vi "Agilent 34401 Read Single Measurement.vi"() -> ()   [LabVIEW 2013]
doc: "This example shows how to configure a measurement and take a single reading."
uses:
  <vilib>/Utility/error.llb/DialogType.ctl
  <instrlib>/Agilent 34401/Public/Data/Read (Single Point).vi
  <instrlib>/Agilent 34401/Agilent 34401.lvlib
panel:
  in  "Function (0: DC Voltage)":u16(ring) items=["DC Voltage", "AC Voltage", "2 - Wire Resistance", "4 - Wire Resistance", "DC Current", "AC Current", "Frequency", "Period", "Continuity", "Diode Checking", "VDC:VDC Ratio", "Temperature", "Capacitance"]
  in  "Enable Auto Range (T: Enable)":bool=TRUE
  in  "Manual Resolution (5.5 Digits)":dbl(ring)=5.5 items=["4.5"=4.5, "5.5"=5.5, "6.5"=6.5]
  in  "Manual Range (1.00)":dbl=1.0 format="%_3f"
  in  "Serial Configuration":T1={"Baud Rate"=9600, "Parity"=2, "Data Bits"=7} {"Data Bits" items=["7"=7, "8"=8]; "Parity" items=["None", "Odd", "Even"]; "Baud Rate" items=["300"=300, "600"=600, "1200"=1200, "2400"=2400, "4800"=4800, "9600"=9600, "19200"=19200]}
  out "Measurement":dbl
  in  "VISA resource name":refnum<visa-resource-name>
  # "(c) 2005-2008 National Instruments.  ALL RIGHTS RESERVED."
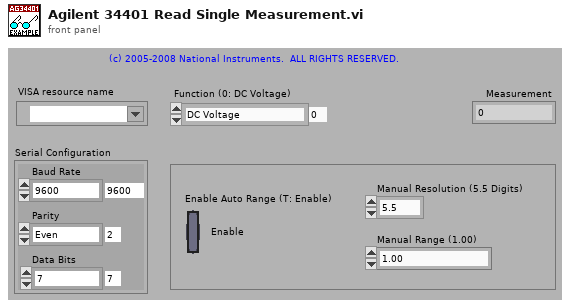
[diagram p1: front panel]
types:
  T1 = cluster{"Baud Rate":u32, "Parity":u16, "Data Bits":u16}
  T2 = typedef "DialogType.ctl" = u16
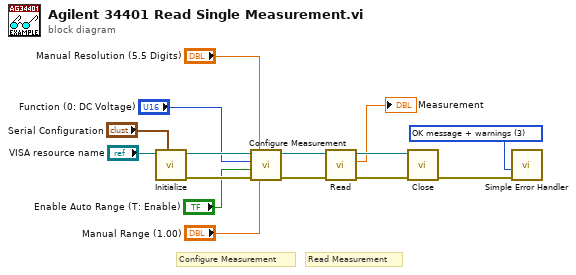
[diagram p0: block diagram]
diagram:
  w1 = T2 3 items=["no dialog", "OK message", "continue or stop message", "OK message + warnings", "continue/stop + warnings"] ("type of dialog (OK msg:1)")
  # "Read Measurement"
  # "Configure Measurement"
  n1 = call <instrlib>:"Initialize.vi"("Serial Configuration"="Serial Configuration", "VISA resource name"="VISA resource name") -> ("error out"=w6:errorcluster, "VISA resource name out"=w7:refnum<visa-resource-name>)  [unwired: 8 in]
  n2 = call <instrlib>:"Configure Measurement.vi"("Manual Range (1.00)"="Manual Range (1.00)", "Manual Resolution (5.5 Digits)"="Manual Resolution (5.5 Digits)", "error in (no error)"=w6, "Enable Auto Range (T: Enable)"="Enable Auto Range (T: Enable)", "Function (0: DC Voltage)"="Function (0: DC Voltage)", "VISA resource name"=w7) -> ("error out"=w8:errorcluster, "VISA resource name out"=w9:refnum<visa-resource-name>)  [unwired: 4 in]
  n3 = call-poly <instrlib>:"Read.vi"("error in (no error)"=w8, "VISA resource name"=w9) -> ("error out"=w12:errorcluster, "Measurement"=→"Measurement":dbl, "VISA resource name out"=w11:refnum<visa-resource-name>)  [unwired: 7 in]
  n4 = call <instrlib>:"Close.vi"("error in (no error)"=w12, "VISA resource name"=w11) -> ("error out"=w15:errorcluster)  [unwired: 9 in]
  n5 = call <vilib>:"Simple Error Handler.vi"("type of dialog (OK msg:1)"=w1, "error in (no error)"=w15) -> ()  [unwired: 3 in, 5 out]
